vi "PID Sine Wave w Enum.vi"() -> ()   [LabVIEW 2017]
uses:
  <vilib>/addons/control/pid/pid.llb/PID (DBL).vi
  <vilib>/addons/control/pid/NI_PID_pid.lvlib
panel:
  out "Counter Value 2":i32
  in  "Enum":enum16{"0", "2000", "4000", "6000"}(ring)=enum."2000"
  in  "Stop VI":bool
  out "Counter Value":i32(graph)
  in  "PID gains":T1={"proportional gain (Kc)"=1.0, "integral time (Ti, min)"=0.01, "derivative time (Td, min)"=0.0} {"derivative time (Td, min)" format="%.3f"; "integral time (Ti, min)" format="%.3f"; "proportional gain (Kc)" format="%.3f"}
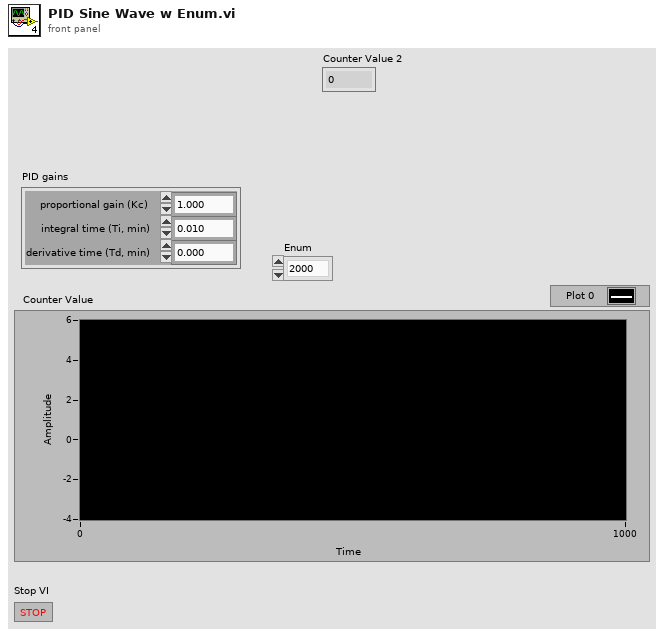
[diagram p1: front panel]
types:
  T1 = cluster{"proportional gain (Kc)":dbl, "integral time (Ti, min)":dbl, "derivative time (Td, min)":dbl}
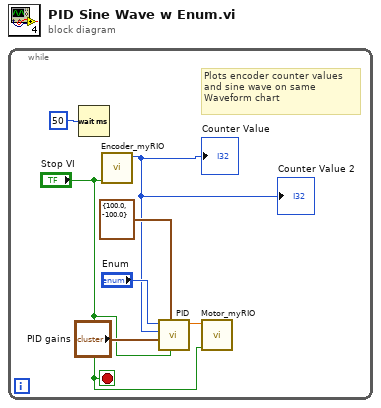
[diagram p0: block diagram]
diagram:
  n1 = while {
    stop <- "Stop VI" stop-if-true
    # "Plots encoder counter values \nand sine wave on same \nWaveform chart"
    n2 = Wait (ms)(milliseconds to wait=u32 50) -> ()  [unwired: 1 out]
    n3 = call "Encoder_myRIO.vi"("Reset"="Stop VI") -> ("Counter Value"=w1:i32)  [unwired: 8 in, 1 out]
    "Counter Value" <- w1
    "Counter Value 2" <- w1
    n4 = call-poly <vilib>:"PID.vi"("reinitialize? (F)"="Stop VI", "output range"=cluster{"output high":dbl, "output low":dbl} {"output high"=100.0, "output low"=-100.0}, "PID gains"="PID gains", "process variable"=w1, "setpoint"="Enum") -> ("output"=w4:dbl)  [unwired: 5 in, 1 out]
    n5 = call "Motor_myRIO.vi"("Stop VI"="Stop VI", "Duty Cycle (-100 to +100)"=w4) -> ()  [unwired: 10 in]
  }
